vi "TCP Close.vi"(8 "Error In":errorcluster, 11 "LINX Decice Config":T1) -> (0 "Error Out":errorcluster, 3 "LINX Decice Config":T1)   [LabVIEW 2020, in "Device.lvlib"]
uses:
  Device.lvlib
  Type Defs/LINX Device Config.ctl
  Type Defs/Interface.ctl
  Type Defs/TCP Config.ctl
  Type Defs/Channels.ctl
  LMH-LINX.lvlib
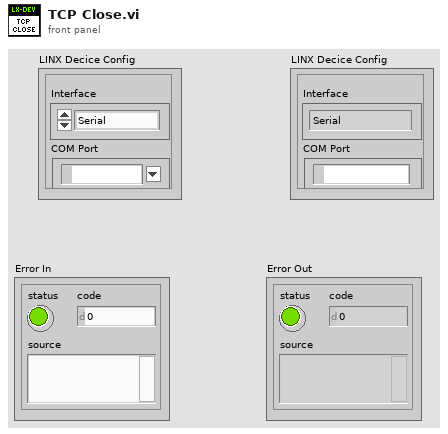
[diagram p1: front panel]
types:
  T1 = typedef "Device.lvlib/LINX Device Config.ctl" = cluster{"Interface":T2, "COM Port":refnum<visa-resource-name>, "TCP Configuration":T3, "Device Family":u8, "Device ID":u8, "Device Name":string, "TCP Ref":refnum<k5>, "Channels":T4}
  T2 = typedef "LMH-LINX.lvlib/Interface.ctl" = enum16{"Serial", "TCP"}
  T3 = typedef "Device.lvlib/TCP Config.ctl" = cluster{"IP Address":string, "Port":u16}
  T4 = typedef "LMH-LINX.lvlib/Channels.ctl" = cluster{"DI":u8[], "DO":u8[], "AI":u8[], "AO":u8[], "PWM":u8[], "QE":u8[], "UART":u8[], "I2C 2":u8[], "SPI":u8[], "CAN":u8[], "Servo":u8[], "AI Ref (V)":dbl, "AI Resolution (Bits)":u8, "AO Ref (V)":dbl, "AO Resolution (Bits)":u8}
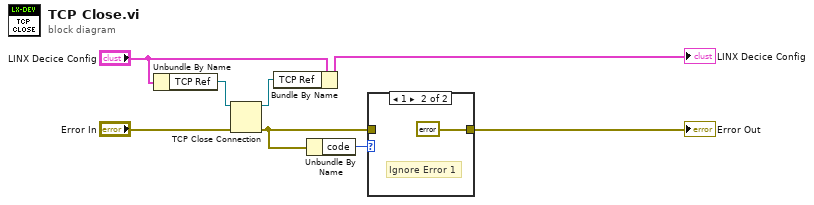
[diagram p0: block diagram]
diagram:
  n1 = Unbundle By Name("LINX Decice Config") -> ("TCP Ref"=w8:refnum<k5>)
  n2 = TCP Close Connection(connection ID=w8, error in (no error)="Error In") -> (connection ID out=w6:refnum<k5>, error out=w1:errorcluster)  [unwired: 1 in]
  n3 = Bundle By Name(cluster="LINX Decice Config", "TCP Ref"=w6) -> (→"LINX Decice Config":T1)
  n4 = Unbundle By Name(w1) -> ("code"=w3:i32)
  n5 = case shown="1" w3 {
    tunnel: [w9 errorcluster {"status"=FALSE, "code"=0, "source"=""} ("error out")] -> w2
    tunnel: w1 -> [w9 _]
    frame 0, Default {
    }
    frame 1 {
      # "Ignore Error 1"
    }
  }
  "Error Out" <- w2
